vi "etc_XCITE_ScanDevices.vi"(8 "error in (no error)":errorcluster {"code" format="%x"}) -> (0 "error out":errorcluster {"code" format="%x"}, 1 "buf_len_out":u32, 2 "ErrorMessage":i32 format="%x", 3 "ph out":u64[](array[numeric]))   [LabVIEW 2019, in "XCite.lvlib"]
doc: "Scans available ports for ETC X-cite devices, and returns a list of handles to devices."
uses:
  XCite.lvlib
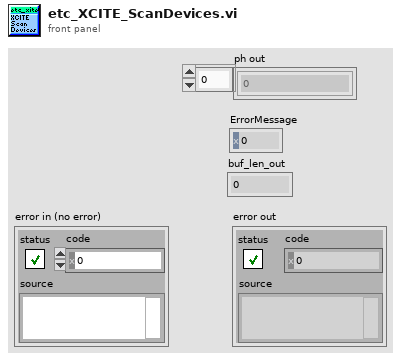
[diagram p1: front panel]
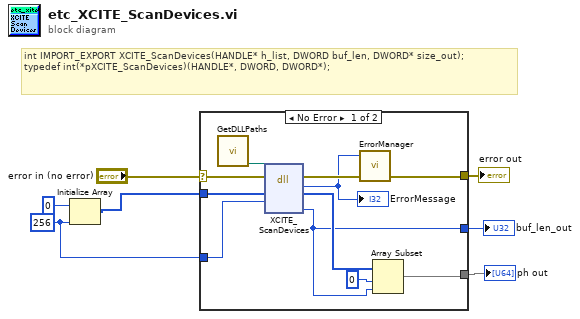
[diagram p0: block diagram]
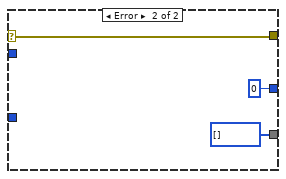
[diagram p2: hidden frame]
diagram:
  w3 = u32 256 ("dimension size")
  # "int IMPORT_EXPORT XCITE_ScanDevices(HANDLE* h_list, DWORD buf_len, DWORD* size_out);\ntypedef int(*pXCITE_ScanDevices)(HANDLE*, DWORD, DWORD*);"
  n1 = Initialize Array(u64 0, w3) -> (w2:u64[])
  n2 = case shown="No Error" "error in (no error)" {
    selector: "error in (no error)" -> [w18 w21]
    tunnel: [w16 w21] -> w7
    tunnel: w2 -> [w14 _]
    tunnel: [w9 u64[] []] -> w5
    tunnel: w3 -> [w12 _]
    tunnel: [w8 u32 0 ("buf_len")] -> w1
    frame No Error {
      n3 = call "GetDLLPaths.vi"() -> ("etc_xcite_path"=w13:path)  [unwired: 8 in, 3 out]
      n4 = dll-call lib="C:/LabVIEWDevFall2024/pco.labview/labview_sdk/runtime/bin64/etc_xcite.dll" fn="XCITE_ScanDevices"(path in=w13, error in=w18, "hlist"=w14, "buf_len"=w12) -> (error out=w17:errorcluster, "return type"=w15:i32, "hlist"=w11:u64[], "size_out"=w8:u32)  [unwired: 3 in, 1 out]
      "ErrorMessage" <- w15
      n5 = call "ErrorManager.vi"("error in (no error)"=w17, "error code"=w15) -> ("error out"=w16:errorcluster)  [unwired: 2 in, 1 out]
      n6 = Array Subset(array=w11, index=0, length=w8) -> (w9:u64[])
    }
    frame Error {
    }
  }
  "error out" <- w7
  "ph out" <- w5
  "buf_len_out" <- w1
